vi "dfd_Group Delay_Normalize Spec.vi"(9 "fs [Hz]":dbl=1.0 format="%.2f", 11 "Band":T1[](array[typedef]) {"subband specs"."weight" format="%.2f"}) -> (3 "Normalized Band":T1[](array[typedef]) {"subband specs"."weight" format="%.2f"})   [LabVIEW 2017, in "NI_DigFilter_Design.lvlib"]
uses:
  <vilib>/addons/Digital Filter Design/NI_DigFilter_Design.lvlib
  <vilib>/addons/Digital Filter Design/_GroupDelay.llb/dfd_Group Delay_Band Spec.ctl
  <vilib>/addons/Digital Filter Design/NI_DigFilterLicensed.lvlib
panel:
  # "freq"
  # "group delay"
  # "weight"
  # "freq"
  # "group delay"
  # "weight"
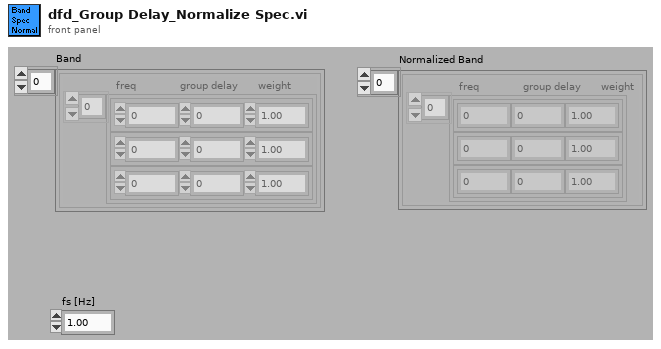
[diagram p1: front panel]
types:
  T1 = typedef "NI_DigFilterLicensed.lvlib/dfd_Group Delay_Band Spec.ctl" = cluster{"subband specs":cluster{"freq":dbl, "group delay":dbl, "weight":dbl}[]}
  T2 = cluster{"freq":dbl, "group delay":dbl, "weight":dbl}[]
  T3 = cluster{"freq":dbl, "group delay":dbl, "weight":dbl}
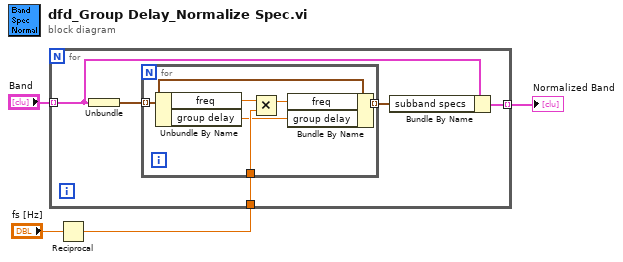
[diagram p0: block diagram]
diagram:
  n1 = Reciprocal(x="fs [Hz]") -> (1/x=w3:dbl)
  n2 = for {
    tunnel: "Band" -> [w7] mode=indexing
    tunnel: w3 -> [w8]
    tunnel: [w5] -> w1 mode=indexing
    n3 = Unbundle(w7) -> ("subband specs"=w9:T2)
    n4 = for {
      tunnel: w9 -> [w15] mode=indexing
      tunnel: w8 -> [w13]
      tunnel: [w12] -> w6 mode=indexing
      n5 = Unbundle By Name(w15) -> ("freq"=w14:dbl, "group delay"=w10:dbl)
      n6 = Multiply(x=w14, y=w13) -> (x*y=w11:dbl)
      n7 = Bundle By Name(cluster=w15, "freq"=w11, "group delay"=w10) -> (w12:T3)
    }
    n8 = Bundle By Name(cluster=w7, "subband specs"=w6) -> (w5:T1)
  }
  "Normalized Band" <- w1
